vi "Close Device Core.vi"(8 "error in (no error)":errorcluster, 11 "IVI_PwrMeter in":refnum<class "IVI_PwrMeter.lvclass">) -> (0 "error out":errorcluster, 3 "IVI_PwrMeter out":refnum<class "IVI_PwrMeter.lvclass">)   [LabVIEW 2016, in "IVI_PwrMeter.lvlib" / "IVI_PwrMeter.lvclass"]
doc: "Close device driver connection."
uses:
  IVI_PwrMeter.lvclass
  IVI_PwrMeter.lvclass/IVI_PwrMeter.ctl
  CSPP_Core/Actors/CS++DeviceActor/CS++DeviceActor.lvclass
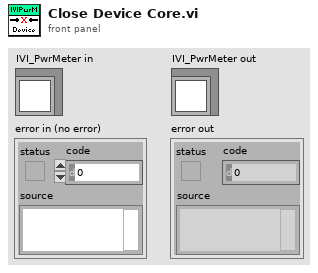
[diagram p1: front panel]
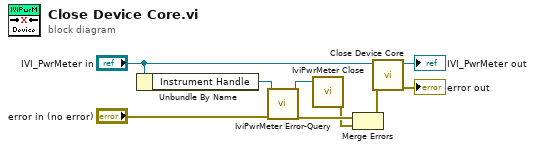
[diagram p0: block diagram]
diagram:
  n1 = Unbundle By Name("IVI_PwrMeter in") -> ("Instrument Handle"=w6:refnum<k15>)
  n2 = call <vilib>:"IviPwrMeter Error-Query.vi"("error in (no error)"="error in (no error)", "instrument handle"=w6) -> ("error out"=w3:errorcluster, "instrument handle out"=w5:refnum<k15>)  [unwired: 6 in, 2 out]
  n3 = call <vilib>:"IviPwrMeter Close.vi"("instrument handle"=w5) -> ("error out"=w2:errorcluster)  [unwired: 10 in]
  n4 = Merge Errors(w3, w2) -> (w1:errorcluster)
  n5 = call-parent "Close Device Core.vi"("error in (no error)"=w1, "CS++DeviceActor in"="IVI_PwrMeter in") -> ("error out"=→"error out":errorcluster, "CS++DeviceActor out"=→"IVI_PwrMeter out":refnum<class "IVI_PwrMeter.lvclass">)  [unwired: 8 in]
